vi "Get FP Status.vi"(9 "View Hierarchy Level":i32, 11 "View Status in":T1) -> (1 "FP Status":T3, 3 "View Status out":T1)   [LabVIEW 2017, in "GUI Views.lvlib" / "GUI Container Actor.lvclass"]
uses:
  GUI Container Actor.lvclass
  typedefs/View Status.ctl
  <vilib>/ActorFramework/Message Enqueuer/Message Enqueuer.lvclass
  typedefs/View Details.ctl
  typedefs/FP Status.ctl
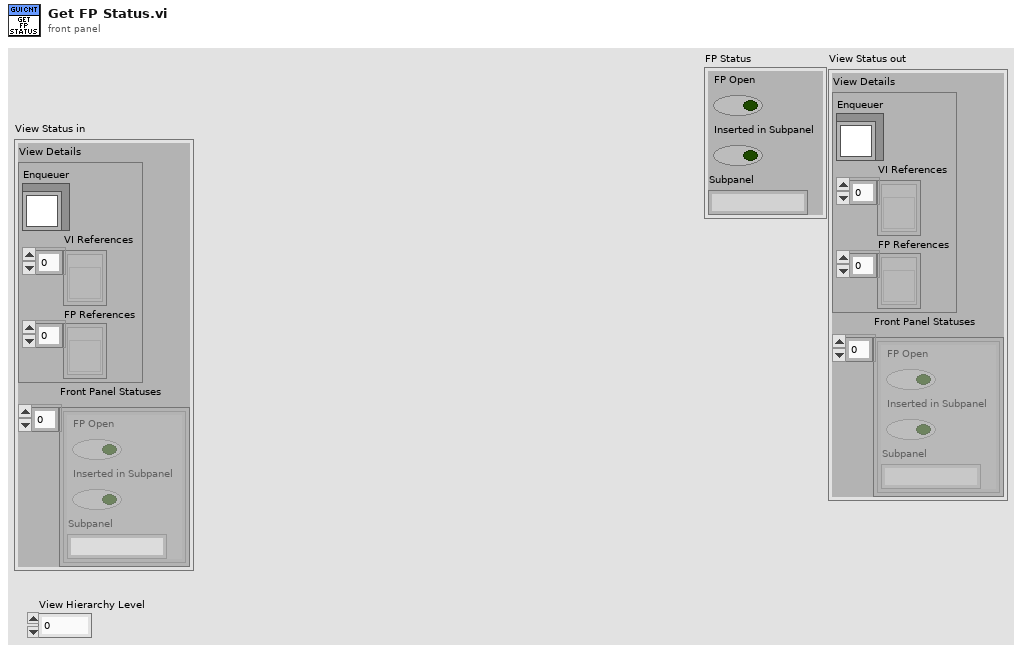
[diagram p1: front panel]
types:
  T1 = typedef "GUI Views.lvlib/GUI Container Actor.lvclass/View Status.ctl" = cluster{"View Details":T2, "Front Panel Statuses":T3[]}
  T2 = typedef "GUI Views.lvlib/GUI Container Actor.lvclass/View Details.ctl" = cluster{"Enqueuer":refnum<class "Message Enqueuer.lvclass">, "VI References":refnum<vi>[], "FP References":refnum<vi>[]}
  T3 = typedef "GUI Views.lvlib/GUI Container Actor.lvclass/FP Status.ctl" = cluster{"FP Open":bool, "Inserted in Subpanel":bool, "Subpanel":string}
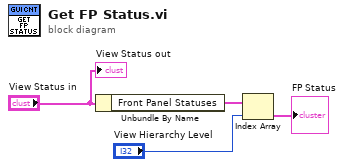
[diagram p0: block diagram]
diagram:
  n1 = Unbundle By Name("View Status in") -> ("Front Panel Statuses"=w3:T3[])
  n2 = Index Array(array=w3, index="View Hierarchy Level") -> (element=→"FP Status":T3)
  "View Status out" <- "View Status in"
